vi "Initialize Attributes.vi"(8 "error in (no error)":errorcluster, 10 "Attribute Data":variant, 11 "CS++PVMonitor in":refnum<class "CS++PVMonitor.lvclass">) -> (0 "error out":errorcluster, 2 "Found?":bool, 3 "CS++PVMonitor out":refnum<class "CS++PVMonitor.lvclass">)   [LabVIEW 2016, in "CS++PVMonitor.lvlib" / "CS++PVMonitor.lvclass"]
doc: "Initialize object attribute.\n\nUnique resources should be allocated elsewhere!"
uses:
  CS++PVMonitor.lvclass
  CS++PVMonitor.lvclass/CS++PVMonitor.ctl
  CS++BaseActor/CS++BaseActor.lvclass
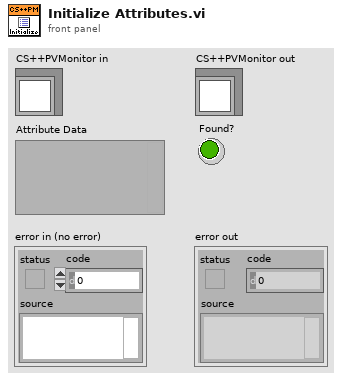
[diagram p1: front panel]
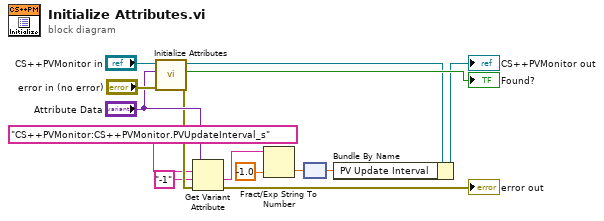
[diagram p0: block diagram]
diagram:
  n1 = call-parent "Initialize Attributes.vi"("error in (no error)"="error in (no error)", "Attribute Data"="Attribute Data", "CS++BaseActor in"="CS++PVMonitor in") -> ("error out"=w10:errorcluster, "Found?"=→"Found?":bool, "CS++BaseActor out"=w6:refnum<class "CS++PVMonitor.lvclass">)  [unwired: 6 in]
  n2 = Get Variant Attribute(Variant="Attribute Data", name="CS++PVMonitor:CS++PVMonitor.PVUpdateInterval_s", default value (empty Variant)="-1", error in=w10) -> (value=w4:string, error out=→"error out":errorcluster)  [unwired: 2 out]
  n3 = Fract/Exp String To Number(string=w4, default (0 dbl)=-1.0) -> (number=w2:dbl)  [unwired: 2 in, 1 out]
  n4 = node(w2) -> (w1:dbl[unit])
  n5 = Bundle By Name(cluster=w6, "PV Update Interval"=w1) -> (→"CS++PVMonitor out":refnum<class "CS++PVMonitor.lvclass">)
